vi "大学核物理实验平台 main.vi"() -> ()   [LabVIEW 2014]
panel:
  out "系统根路径":path
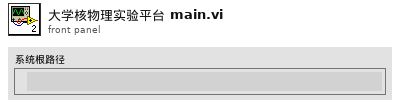
[diagram p1: front panel]
types:
  T1 = enum32{"Invalid", "Standard", "Closed", "Hidden", "Minimized", "Maximized"}
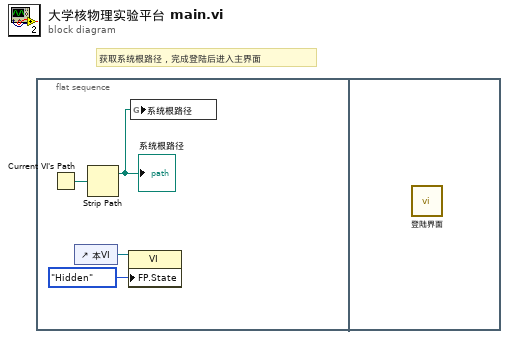
[diagram p0: block diagram]
diagram:
  # "获取系统根路径，完成登陆后进入主界面"
  n1 = flat-sequence {
    frame #0 {
      n2 = Current VI's Path() -> (path=w1:path)
      n3 = control-ref of="本VI"() -> (w3:refnum<vi>)
      n4 = Strip Path(path=w1) -> (stripped path=w2:path)  [unwired: 1 out]
      "系统根路径" <- w2
      n5 = property class="VI"(reference=w3, "FP.State"=T1."Hidden" ("前面板窗口:状态")) -> ()  [unwired: 1 in, 2 out]
      n6 = global write "系统全局变量.vi" "系统根路径"(w2) -> ()
    }
    frame #1 {
      n7 = call "登陆界面.vi"() -> ()  [unwired: 12 in]
    }
  }
